vi "Loginoff.vi"() -> ()   [LabVIEW 2017]
panel:
  in  "Tab Control":enum32{"Page 1", "Page 2"}(tab)
  in  "Enter":bool
  in  "Username":string
  in  "Password":string
  in  "Close":bool
  in  "Login":bool
  in  "Reset":bool
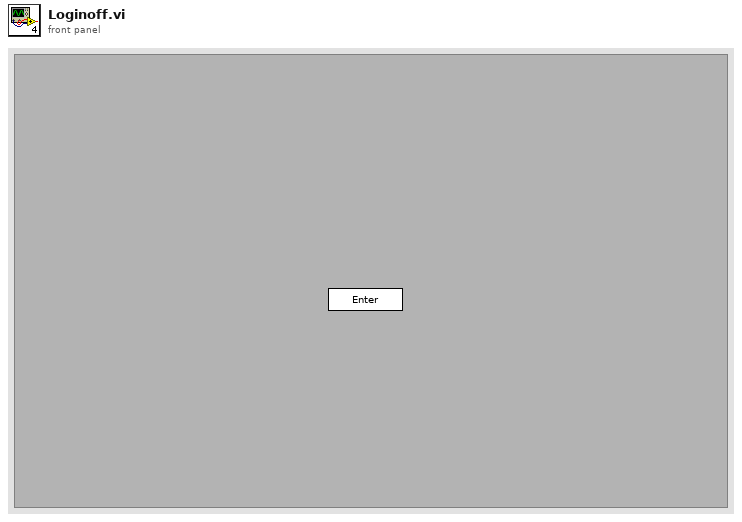
[diagram p1: front panel]
types:
  T1 = enum32{"Invalid", "Standard", "Closed", "Hidden", "Minimized", "Maximized"}
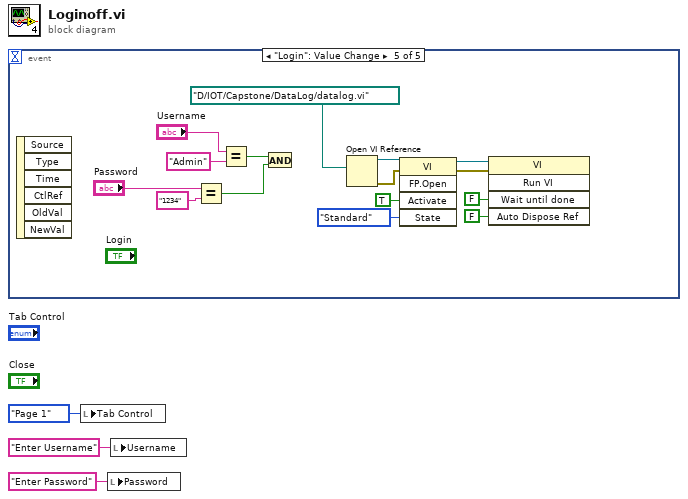
[diagram p0: block diagram]
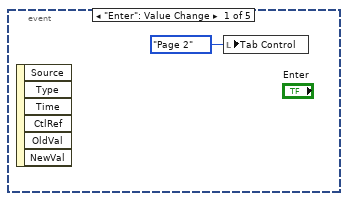
[diagram p2: hidden frame]
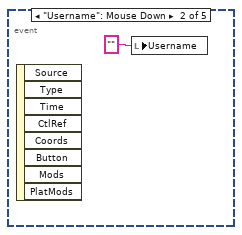
[diagram p3: hidden frame]
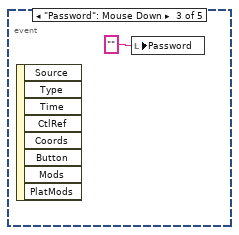
[diagram p4: hidden frame]
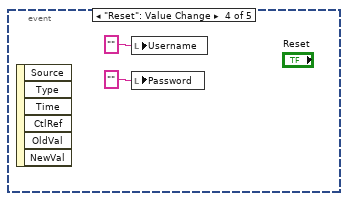
[diagram p5: hidden frame]
diagram:
  n1 = event shown="[4] \"Login\": Value Change" {
    selector: _ -> [_ _ _ _ _]
    dyn-events: _ -> [_ _ _ _ _]
    timeout: _ -> [_ _ _ _ _]
    event "Enter": Value Change {
      n2 = event-data() -> ()  [unwired: 1 in, 6 out]
      n3 = local write "Tab Control"(enum32{"Page 1", "Page 2"}."Page 2" ("Tab Control")) -> ()
    }
    event "Username": Mouse Down {
      n4 = event-data() -> ()  [unwired: 1 in, 8 out]
      n5 = local write "Username"("" ("Username")) -> ()
    }
    event "Password": Mouse Down {
      n6 = event-data() -> ()  [unwired: 1 in, 8 out]
      n7 = local write "Password"("" ("Password")) -> ()
    }
    event "Reset": Value Change {
      n8 = event-data() -> ()  [unwired: 1 in, 6 out]
      n9 = local write "Username"("" ("Username")) -> ()
      n10 = local write "Password"("" ("Password")) -> ()
    }
    event "Login": Value Change {
      n11 = event-data() -> ()  [unwired: 1 in, 6 out]
      n12 = Equal?(x="Password", y="1234") -> (x = y?=w18:bool)
      n13 = Equal?(x="Username", y="Admin") -> (x = y?=w19:bool)
      n14 = And(x=w19, y=w18) -> ()  [unwired: 1 out]
      n15 = Open VI Reference(vi path=path "D:/IOT/Capstone/DataLog/datalog.vi") -> (vi reference=w16:refnum<vi>, error out=w15:errorcluster)  [unwired: 5 in]
      n16 = invoke class="VI" method="FP.Open"(reference=w16, error in=w15, "Activate"=TRUE ("Activate?"), "State"=T1."Standard") -> (reference out=w14:refnum<vi>, error out=w13:errorcluster)  [unwired: 1 in, 3 out]
      n17 = invoke class="VI" method="Run VI"(reference=w14, error in=w13, "Wait until done"=FALSE ("Wait Until Done"), "Auto Dispose Ref"=FALSE ("Auto Dispose Reference")) -> ()  [unwired: 1 in, 5 out]
    }
  }
  n18 = local write "Tab Control"(enum32{"Page 1", "Page 2"}."Page 1" ("Tab Control")) -> ()
  n19 = local write "Password"("Enter Password" ("Password")) -> ()
  n20 = local write "Username"("Enter Username" ("Username")) -> ()
